vi "Cookies from Header Value.vi"(8 "error in (no error)":errorcluster, 11 "Cookie Header Value":string) -> (0 "error out":errorcluster, 3 "Cookies":refnum<class "Cookie.lvclass">[](array[class]))   [LabVIEW 2020, in "HTTP Utils.lvlib" / "Cookie.lvclass"]
uses:
  Cookie.lvclass
  Cookie.lvclass/Cookie.ctl
  HTTP Utils.lvlib
  lv-uri/URI/URI.lvlib
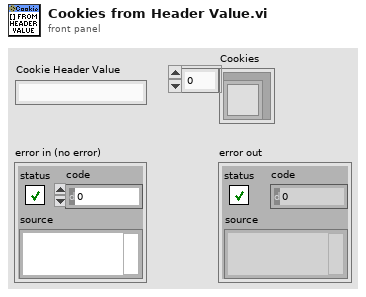
[diagram p1: front panel]
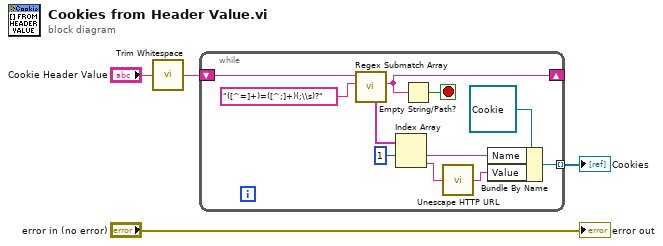
[diagram p0: block diagram]
diagram:
  n1 = call <vilib>:"Trim Whitespace.vi"("string"="Cookie Header Value") -> ("trimmed string"=w2:string)  [unwired: 1 in]
  n2 = while {
    shift-right: [w11] -> _
    shift-left: w2 -> [w15]
    tunnel: [w7] -> w1 mode=indexing
    stop <- w10 stop-if-true
    n3 = call "Regex Submatch Array.vi"("regular expression"="([^=]+)=([^;]+)(;\\s)?", "string"=w15) -> ("after match"=w11:string, "matches"=w13:string[])  [unwired: 5 in, 3 out]
    n4 = Index Array(array=w13, index #1=1 ("index")) -> (element #1=w8:string, element #2=w6:string)  [unwired: 1 in]
    n5 = Empty String/Path?(string/path=w11) -> (empty?=w10:bool)
    n6 = call "Unescape HTTP URL.vi"("escaped string in"=w6) -> ("unescaped string out"=w5:string)
    n7 = Bundle By Name(cluster=refnum<class "Cookie.lvclass"> refnum ("HTTP Utils.lvlib:Cookie.lvclass"), "Name"=w8, "Value"=w5) -> (w7:refnum<class "Cookie.lvclass">)
  }
  "Cookies" <- w1
  "error out" <- "error in (no error)"
